vi "Auton Drive Dictation.vi"(8 "Reset Encoders":bool, 9 "Distance (inches)":dbl=150.0, 10 "Direction (0-359)":dbl, 11 "Speed (0 to 1)":dbl=-0.75) -> (0 "Joy Y":dbl, 1 "Joy X":dbl, 2 "Distance Reached?":bool=TRUE)   [LabVIEW 2014]
uses:
  Begin/Global RefNums.vi
  <vilib>/addons/control/pid/pid.llb/PID (DBL).vi
  <vilib>/addons/control/pid/NI_PID_pid.lvlib
panel:
  out "Counts":i32=789
  in  "PID Range":dbl=7.85398 format="%#_13g"
  in  "PID gains":T1={"proportional gain (Kc)"=0.005, "integral time (Ti, min)"=0.0001, "derivative time (Td, min)"=0.0} {"derivative time (Td, min)" format="%.3f"; "integral time (Ti, min)" format="%.7f"; "proportional gain (Kc)" format="%.3f"}
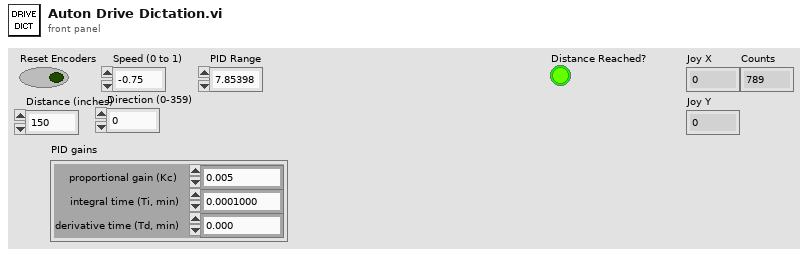
[diagram p1: front panel]
types:
  T1 = cluster{"proportional gain (Kc)":dbl, "integral time (Ti, min)":dbl, "derivative time (Td, min)":dbl}
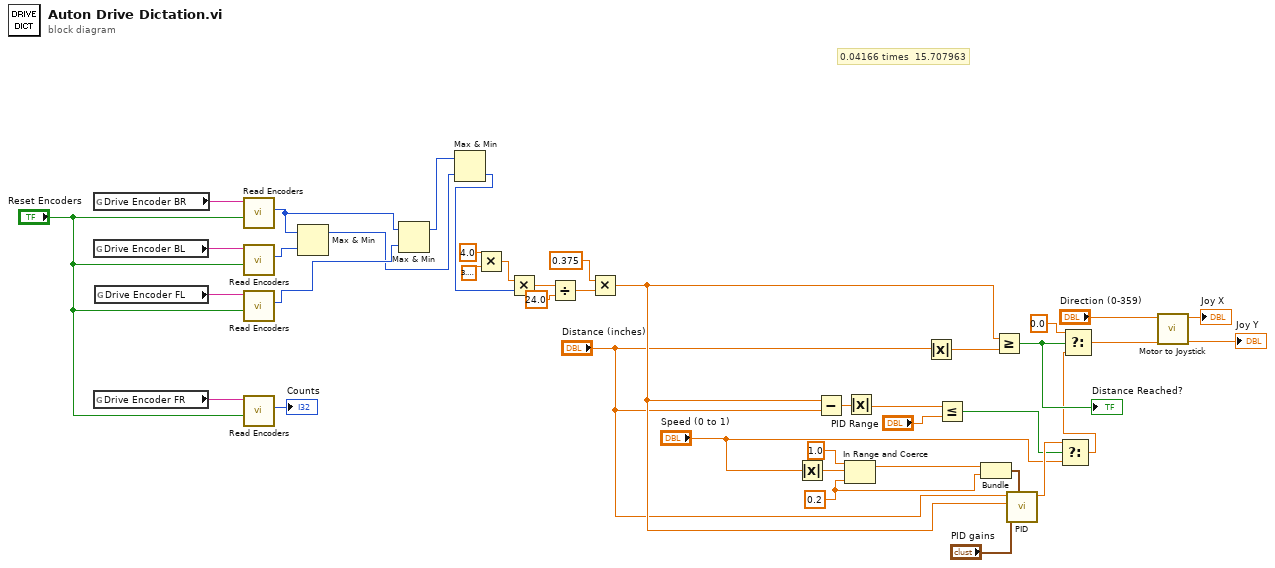
[diagram p0: block diagram]
diagram:
  w6 = 0.2 ("lower limit")
  # "0.04166 times  15.707963"
  n1 = global read "Global RefNums.vi" "Drive Encoder BR"() -> (w41:string)
  n2 = global read "Global RefNums.vi" "Drive Encoder BL"() -> (w15:string)
  n3 = global read "Global RefNums.vi" "Drive Encoder FR"() -> (w10:string)
  n4 = global read "Global RefNums.vi" "Drive Encoder FL"() -> (w13:string)
  n5 = call "Read Encoders.vi"("Reset Encoders"="Reset Encoders", "Encoder"=w41) -> ("Counts"=w5:i32)  [unwired: 9 in]
  n6 = call "Read Encoders.vi"("Reset Encoders"="Reset Encoders", "Encoder"=w15) -> ("Counts"=w14:i32)  [unwired: 9 in]
  n7 = call "Read Encoders.vi"("Reset Encoders"="Reset Encoders", "Encoder"=w13) -> ("Counts"=w4:i32)  [unwired: 9 in]
  n8 = call "Read Encoders.vi"("Reset Encoders"="Reset Encoders", "Encoder"=w10) -> ("Counts"=→"Counts":i32)  [unwired: 9 in]
  n9 = Max & Min(x=w5, y=w14) -> (max(x,y)=w2:i32)  [unwired: 1 out]
  n10 = Max & Min(x=w5, y=w4) -> (max(x,y)=w3:i32)  [unwired: 1 out]
  n11 = Max & Min(x=w3, y=w2) -> (min(x,y)=w1:i32)  [unwired: 1 out]
  n12 = Multiply(x=4.0, y=3.141592653589793) -> (x*y=w33:dbl)
  n13 = Multiply(x=w33, y=w1) -> (x*y=w32:dbl)
  n14 = Divide(x=w32, y=24.0) -> (x/y=w31:dbl)
  n15 = Multiply(x=0.375 ("y"), y=w31) -> (x*y=w20:dbl)
  n16 = Absolute Value(x="Speed (0 to 1)") -> (abs(x)=w28:dbl)
  n17 = Subtract(x=w20, y="Distance (inches)") -> (x-y=w22:dbl)
  n18 = In Range and Coerce(upper limit=1.0, x=w28, lower limit=w6) -> (coerced(x)=w27:dbl)  [unwired: 1 out]
  n19 = Absolute Value(x=w22) -> (abs(x)=w21:dbl)
  n20 = Absolute Value(x="Distance (inches)") -> (abs(x)=w16:dbl)
  n21 = Less Or Equal?(x=w21, y="PID Range") -> (x <= y?=w18:bool)
  n22 = Bundle("upper limit"=w27, "lower limit"=w6) -> (w7:cluster{"upper limit":dbl, "lower limit":dbl})  [unwired: 1 in]
  n23 = Greater Or Equal?(x=w20, y=w16) -> (x >= y?=w40:bool)
  "Distance Reached?" <- w40
  n24 = call-poly <vilib>:"PID.vi"("output range"=w7, "PID gains"="PID gains", "process variable"=w20, "setpoint"="Distance (inches)") -> ("output"=w25:dbl)  [unwired: 6 in, 1 out]
  n25 = Select(t=w25, s=w18, f="Speed (0 to 1)") -> (s? t:f=w23:dbl)
  n26 = Select(t=0.0, s=w40, f=w23) -> (s? t:f=w38:dbl)
  n27 = call "Motor to Joystick.vi"("Drive Motor"=w38, "Rotational Motor"="Direction (0-359)") -> ("Joy Y"=→"Joy Y":dbl, "Joy X"=→"Joy X":dbl)  [unwired: 8 in]
